vi "Configure Dialog.vi"(8 "error in (no error)":errorcluster, 11 "Set Delays Msg.lvclass":refnum<class "Set Delays Msg.lvclass">) -> (0 "error out":errorcluster, 2 "Ok?":bool, 3 "Set Delays Msg.lvclass":refnum<class "Set Delays Msg.lvclass">)   [LabVIEW 2020, in "BNT_ULx.lvlib" / "Set Delays Msg.lvclass"]
uses:
  Set Delays Msg.lvclass
  Set Delays Msg.lvclass/Set Delays Msg.ctl
panel:
  in  "Start Index":i32
  in  "PWM Delays":dbl[](array[numeric]) format="%.3g"
  in  "Cancel Button":bool
  in  "OK Button":bool
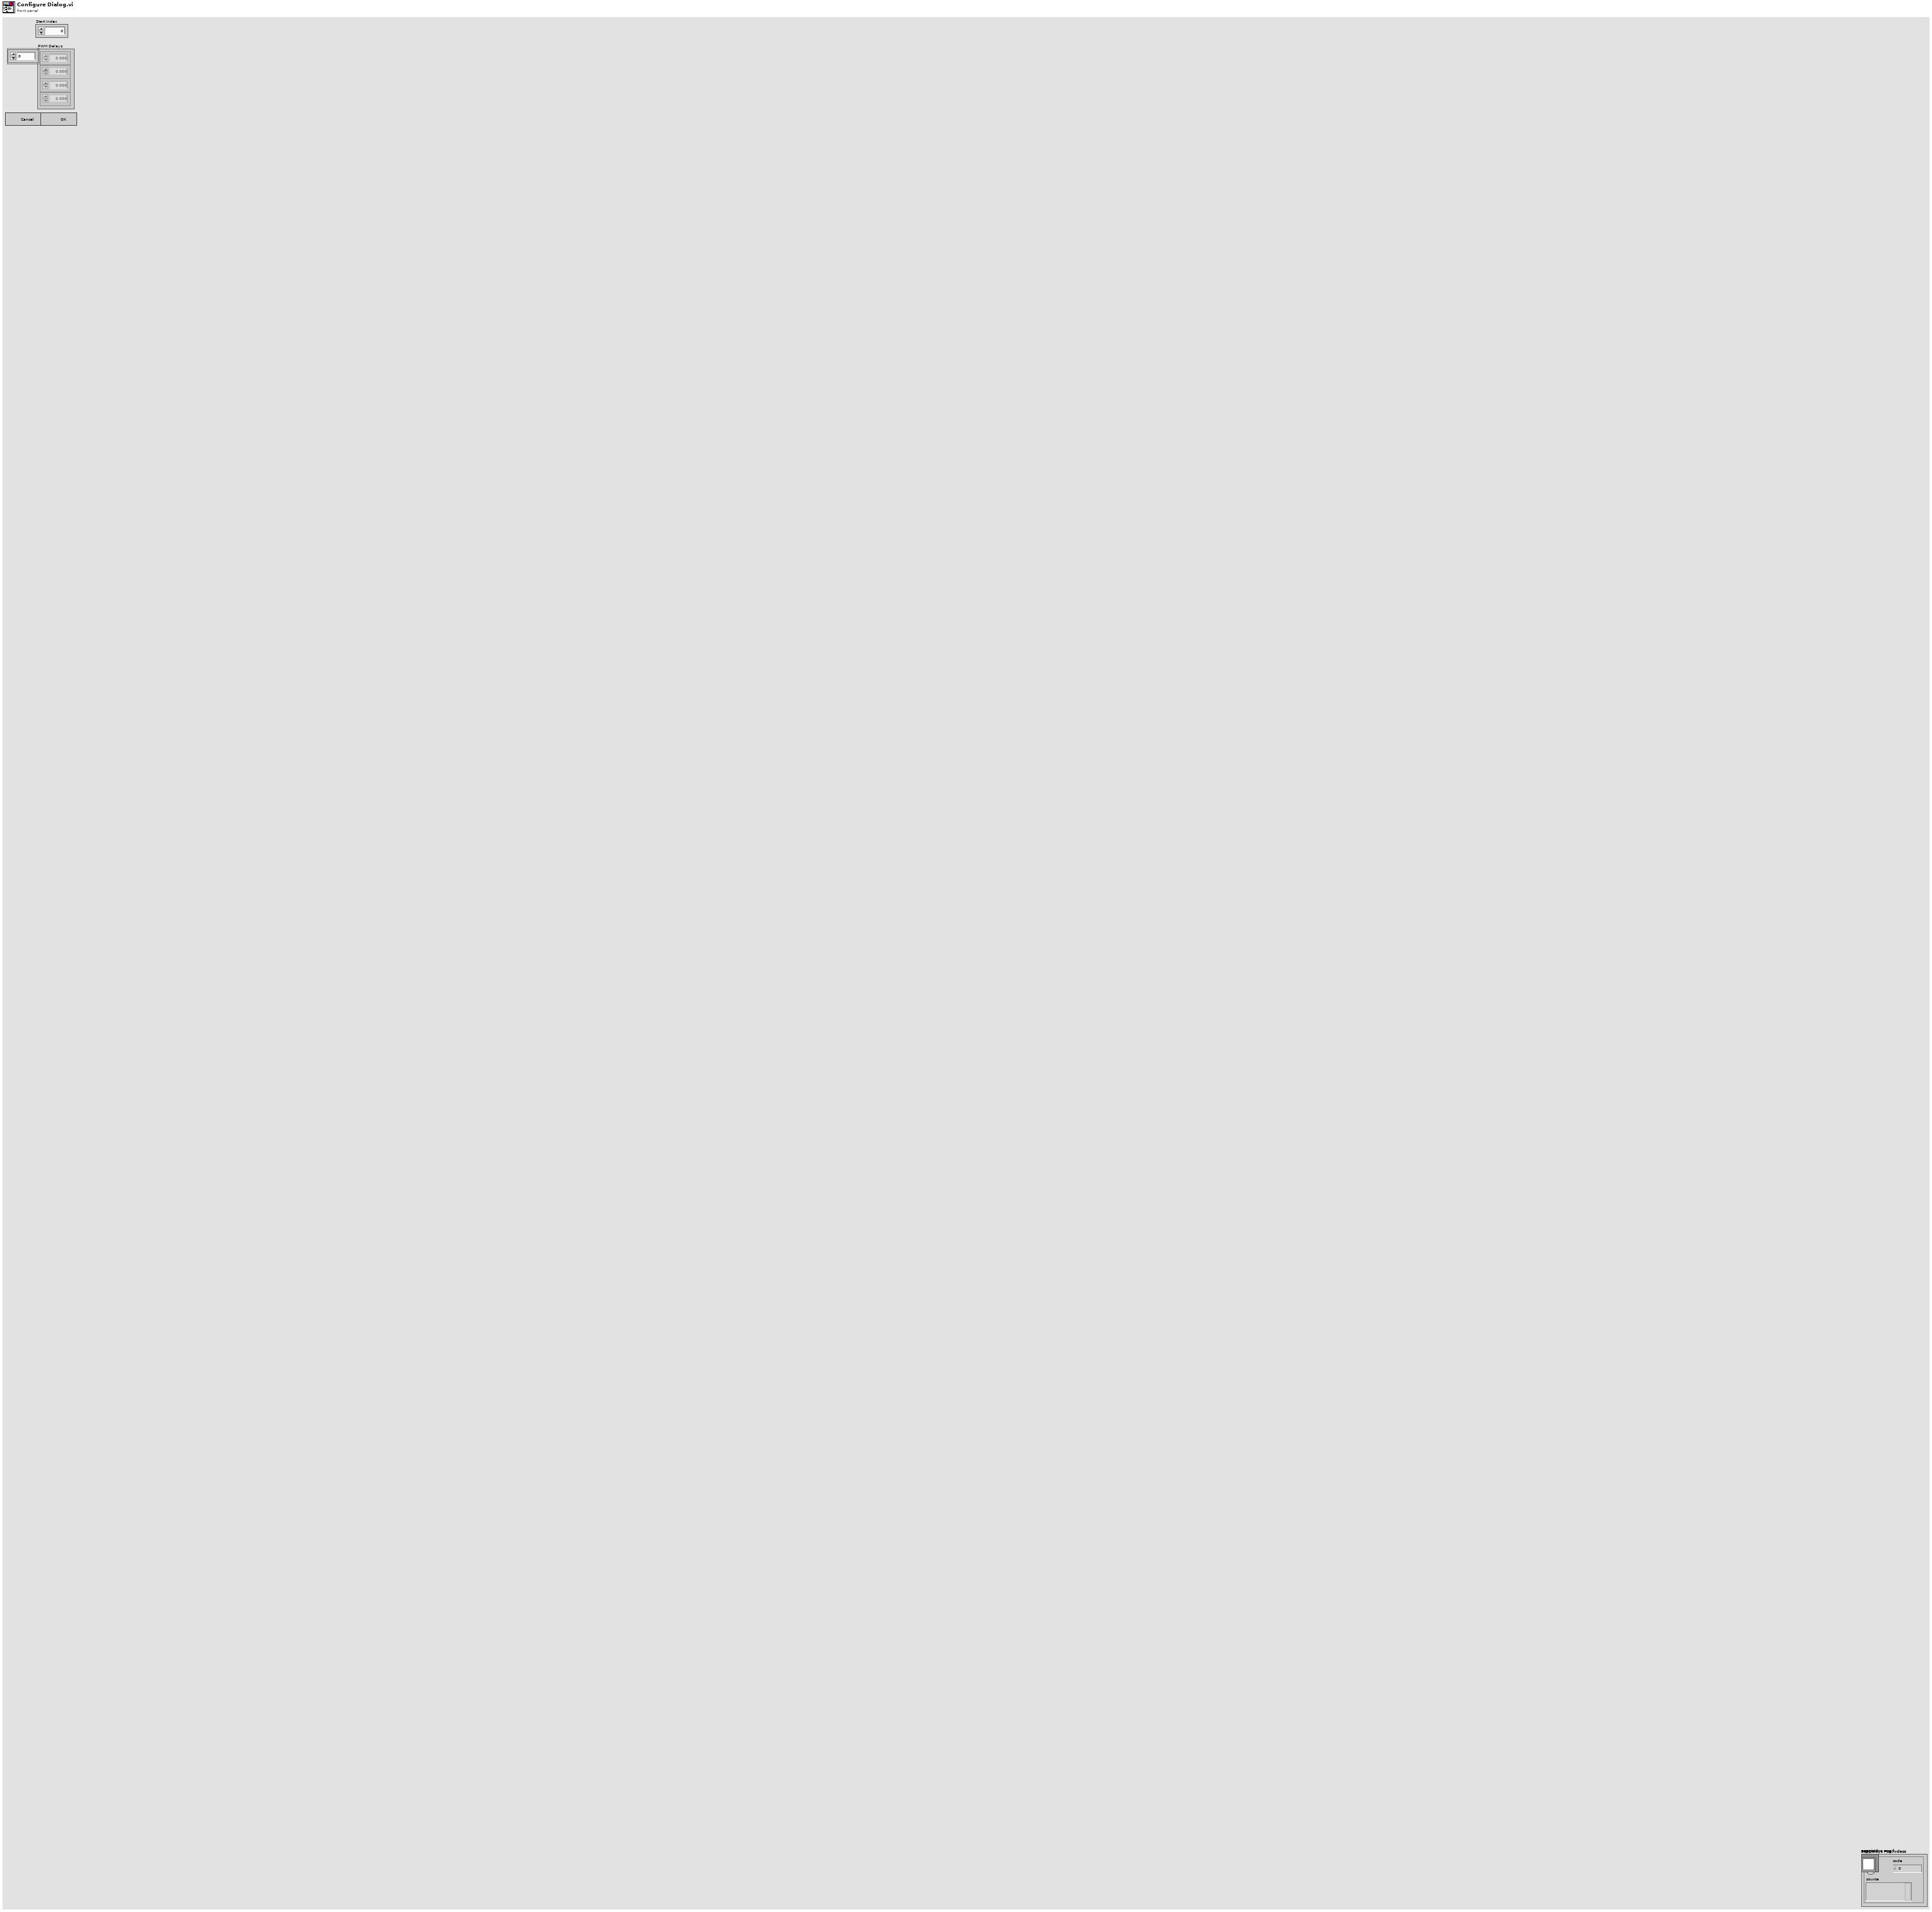
[diagram p1: front panel]
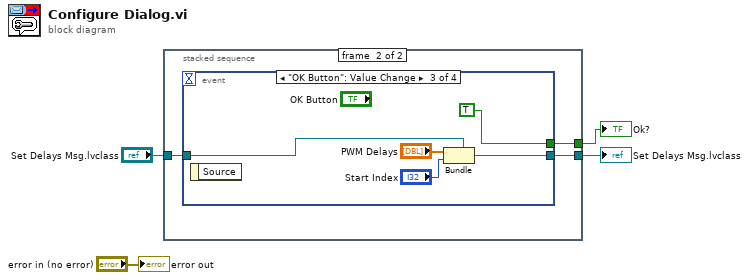
[diagram p0: block diagram]
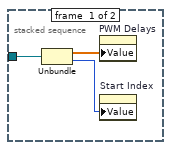
[diagram p2: hidden frame]
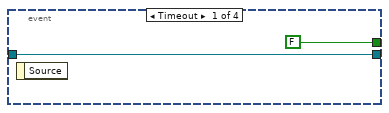
[diagram p3: hidden frame]
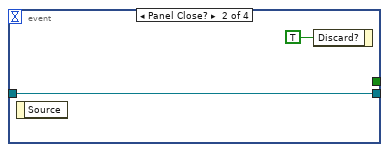
[diagram p4: hidden frame]
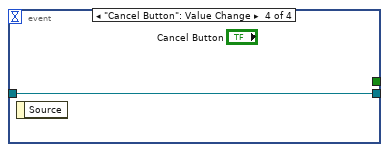
[diagram p5: hidden frame]
diagram:
  n1 = stacked-sequence {
    tunnel: [_ w10] -> w3
    tunnel: [_ w9] -> w2
    tunnel: "Set Delays Msg.lvclass" -> [w7 w8]
    frame #0 {
      n2 = Unbundle ("Seq0Unbundler")(w7) -> (w6:dbl[], w5:i32)
      n3 = property on="PWM Delays" class="Arr (strict)"("Value"=w6) -> ()  [unwired: 2 in, 2 out]
      n4 = property on="Start Index" class="DigNum (strict)"("Value"=w5) -> ()  [unwired: 2 in, 2 out]
    }
    frame #1 {
      n5 = event shown="[2] \"OK Button\": Value Change" {
        selector: _ -> [_ _ _ _]
        dyn-events: _ -> [_ _ _ _]
        timeout: _ -> [_ _ _ _]
        tunnel: [w11 w13 w17 w20] -> w9
        tunnel: w8 -> [w11 w13 w19 w20]
        tunnel: [FALSE _ TRUE _] -> w10
        event Timeout {
          n6 = event-data() -> ()  [unwired: 1 in, 1 out]
        }
        event Panel Close? {
          n7 = event-data() -> ()  [unwired: 1 in, 1 out]
          n8 = event-data ("Event Filter Node")("Discard?"=TRUE) -> ()  [unwired: 1 in, 1 out]
        }
        event "OK Button": Value Change {
          n9 = event-data() -> ()  [unwired: 1 in, 1 out]
          n10 = Bundle ("Main-Bundler")(cluster=w19, "PWM Delays", "Start Index") -> (w17:refnum<class "Set Delays Msg.lvclass">)
        }
        event "Cancel Button": Value Change {
          n11 = event-data() -> ()  [unwired: 1 in, 1 out]
        }
      }
    }
  }
  "Ok?" <- w3
  "Set Delays Msg.lvclass" <- w2
  "error out" <- "error in (no error)"
